vi "calculate.vi"(8 "error in (no error)":errorcluster, 10 "Numbers.lvclass":refnum<class "Numbers.lvclass">, 11 "Add in":refnum<class "Add.lvclass">) -> (0 "error out":errorcluster, 3 "Add out":refnum<class "Add.lvclass">)   [LabVIEW 2018, in "Add.lvclass"]
uses:
  Add.lvclass
  Numbers Class/Numbers.lvclass
  Numbers Class/Numbers.lvclass/Numbers.ctl
  Add.lvclass/Add.ctl
  ConsoleOut/Print Options.ctl
  Chain Class/Chain.lvclass
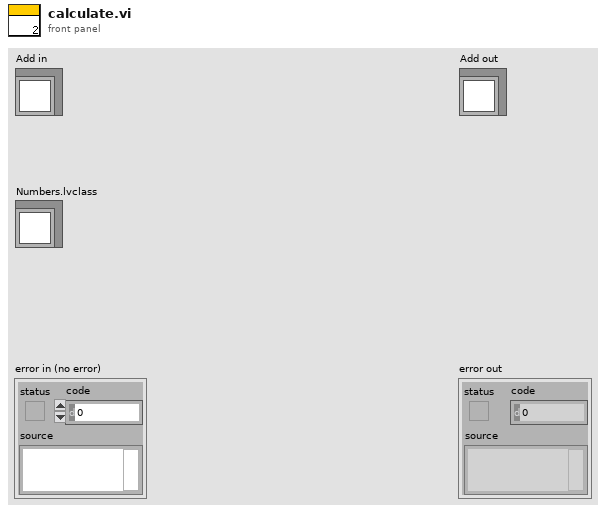
[diagram p1: front panel]
types:
  T1 = typedef "Print Options.ctl" = enum16{"Create", "Get Reference", "Print", "Print Header", "Close"}
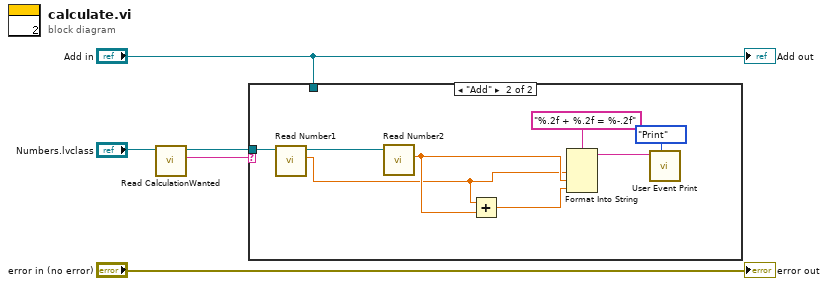
[diagram p0: block diagram]
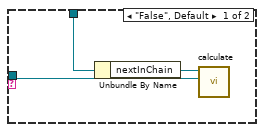
[diagram p2: hidden frame]
diagram:
  n1 = call "Read CalculationWanted.vi"("Numbers in"="Numbers.lvclass") -> ("CalculationWanted"=w3:string, "Numbers out"=w2:refnum<class "Numbers.lvclass">)  [unwired: 8 in, 1 out]
  n2 = case shown="\"Add\"" w3 {
    tunnel: w2 -> [w8 w16]
    tunnel: "Add in" -> [w7 _]
    frame "False", Default {
      n3 = Unbundle By Name(w7) -> ("nextInChain"=w6:refnum<class "Chain.lvclass">)
      n4 = call-dynamic "calculate.vi"("Numbers.lvclass"=w8, "Chain in"=w6) -> ()  [unwired: 8 in, 2 out]
    }
    frame "Add" {
      n5 = call "Read Number1.vi"("Numbers in"=w16) -> ("Number1"=w11:dbl, "Numbers out"=w15:refnum<class "Numbers.lvclass">)  [unwired: 8 in, 1 out]
      n6 = call "Read Number2.vi"("Numbers in"=w15) -> ("Number2"=w12:dbl)  [unwired: 8 in, 2 out]
      n7 = Add(x=w11, y=w12) -> (x+y=w13:dbl)
      n8 = Format Into String(format string="%.2f + %.2f = %-.2f", w11, w12, w13) -> (resulting string=w10:string)  [unwired: 2 in, 1 out]
      n9 = call "User Event Print.vi"("Options"=Print_Options."Print", "String to Print"=w10) -> ()  [unwired: 8 in, 2 out]
    }
  }
  "error out" <- "error in (no error)"
  "Add out" <- "Add in"
